vi "ATF-Storage NS Read Data.vi"(8 "error in (no error)":errorcluster, 9 "data":string, 10 "Queues.R ER Storage":refnum<queue>, 11 "Notifier in":refnum<notifier>) -> (0 "error out":errorcluster)   [LabVIEW 2022 SP3]
uses:
  Storage cRIO/RT Controls/ATF Storage-Data Type Control screen.ctl
  Controls/SeCrTs-NS Data type.ctl
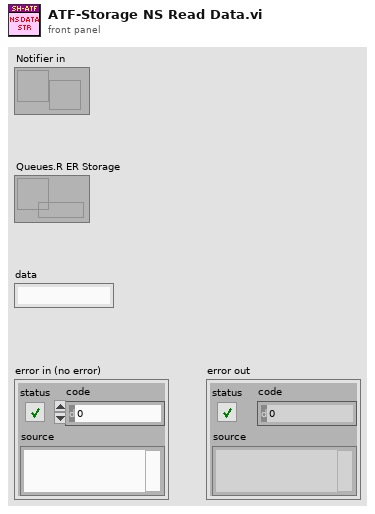
[diagram p1: front panel]
types:
  T1 = typedef "ATF Storage-Data Type Control screen.ctl" = cluster{"DI_Data":digitalwaveform[], "Drive_A_C":waveform(dbl)[], "Drive_A_D":waveform(dbl)[], "Drive_L_C":waveform(dbl)[], "Drive_L_D":waveform(dbl)[], "Loop Status":bool[], "CDT Timer":dbl, "RT Error":cluster{"Error Code":string, "Error Source":string}, "DO":waveform(dbl)[], "SEQ Monitor":string[], "Device List":string}
  T2 = cluster{"Error Code":string, "Error Source":string}
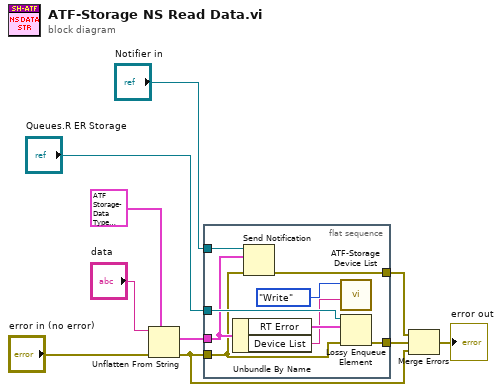
[diagram p0: block diagram]
diagram:
  n1 = Unflatten From String(type=T1 {"DI_Data"=[], "Drive_A_C"=[], "Drive_A_D"=[], "Drive_L_C"=[], "Drive_L_D"=[], "Loop Status"=[], "CDT Timer"=0.0, "RT Error"={"Error Code"="", "Error Source"=""}, "DO"=[], "SEQ Monitor"=[], "Device List"=""} ("Cluster"), binary string="data", error in (no error)="error in (no error)") -> (value=w6:T1, error out=w4:errorcluster)  [unwired: 2 in, 1 out]
  n2 = flat-sequence {
    tunnel: "Notifier in" -> [w19]
    tunnel: "Queues.R ER Storage" -> [w18]
    tunnel: w6 -> [w14]
    tunnel: w4 -> [w13]
    tunnel: [w12] -> w3
    tunnel: [w11] -> w2
    frame #0 {
      n3 = Unbundle By Name(w14) -> ("RT Error"=w17:T2, "Device List"=w15:string)
      n4 = Send Notification(notification=w14, notifier=w19, error in (no error)=w13) -> (error out=w12:errorcluster)  [unwired: 1 out]
      n5 = call "ATF-Storage Device List.vi"("DL"=w15, "Enum"=enum16{"Read", "Write", "Clear"}."Write") -> ()  [unwired: 9 in, 1 out]
      n6 = Lossy Enqueue Element(queue=w18, element=w17, error in (no error)=w13) -> (error out=w11:errorcluster)  [unwired: 3 out]
    }
  }
  n7 = Merge Errors(w3, w2, w4) -> (→"error out":errorcluster)
